vi "FFOvl.vi"() -> (0 "FFOvl":u8)   [LabVIEW 2015]
uses:
  ESLSCDLL.dll
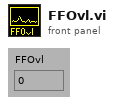
[diagram p1: front panel]
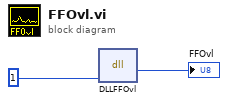
[diagram p0: block diagram]
diagram:
  n1 = dll-call lib="C:/ENTW/PCIE/64bit/lv64/1cam/board.vis/ESLSCDLL.dll" fn="DLLFFOvl"("drv"=u32 1) -> ("Rückgabetyp"=→"FFOvl":u8)  [unwired: 4 in, 2 out]
